vi "ClassInitFGV.vi"(8 "error in (no error)":errorcluster, 11 "CtlReferences in":refnum<class "CtlReferences.lvclass">) -> (0 "error out":errorcluster, 3 "CtlReferences out":refnum<class "CtlReferences.lvclass">)   [LabVIEW 2020, in "CtlReferences.lvlib" / "CtlReferences.lvclass"]
uses:
  CtlReferences.lvclass
  CtlReferences.lvclass/CtlReferences.ctl
  ctlRef_Maps/ctlRef_Maps.lvclass
  C:/Viviota/Projects/R&D/VIV_ctlReferences/CtlReferences/CtlReferences.lvclass
  C:/Viviota/Projects/R&D/VIV_ctlReferences/ctlRef_Maps/ctlRef_Maps.lvclass
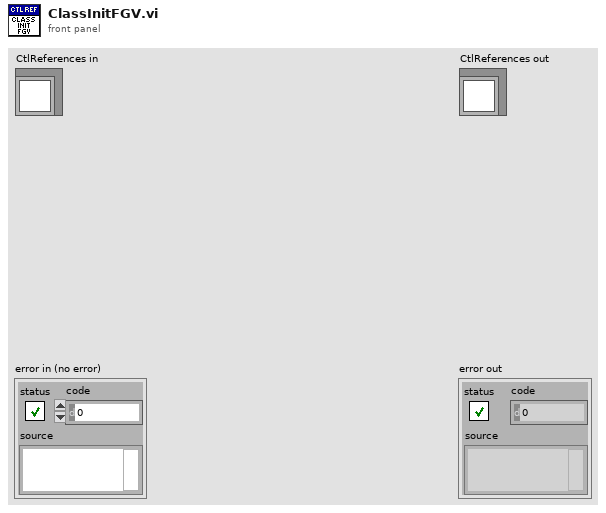
[diagram p1: front panel]
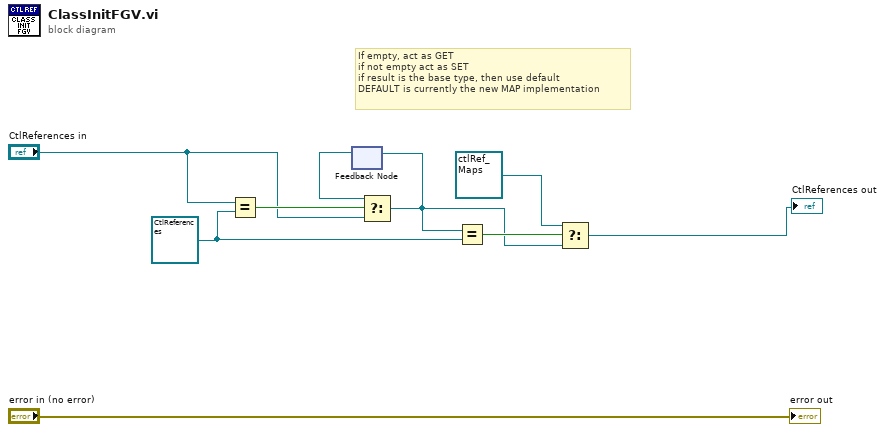
[diagram p0: block diagram]
diagram:
  w5 = refnum<class "CtlReferences.lvclass"> refnum ("CtlReferences in")
  # "If empty, act as GET\nif not empty act as SET\nif result is the base type, then use default\nDEFAULT is currently the new MAP implementation"
  n1 = Equal?(x="CtlReferences in", y=w5) -> (x = y?=w8:bool)
  n2 = feedback #1() -> (w6:refnum<class "CtlReferences.lvclass">)  [unwired: 1 in]
  n3 = Select(t=w6, s=w8, f="CtlReferences in") -> (s? t:f=w3:refnum<class "CtlReferences.lvclass">)
  n4 = feedback-in #1(w3) -> ()
  n5 = Equal?(x=w3, y=w5) -> (x = y?=w4:bool)
  n6 = Select(t=refnum<class "ctlRef_Maps.lvclass"> refnum ("CtlReferences.lvlib:ctlRef_Maps.lvclass"), s=w4, f=w3) -> (s? t:f=→"CtlReferences out":refnum<class "CtlReferences.lvclass">)
  "error out" <- "error in (no error)"
